vi "反控仪器单参数通用.vi"(8 "错误输入（无错误）":errorcluster, 9 "参数":string, 10 "value float":sgl, 11 "chose":string="写入") -> (0 "错误输出":errorcluster, 3 "超时？":bool)   [LabVIEW 2016]
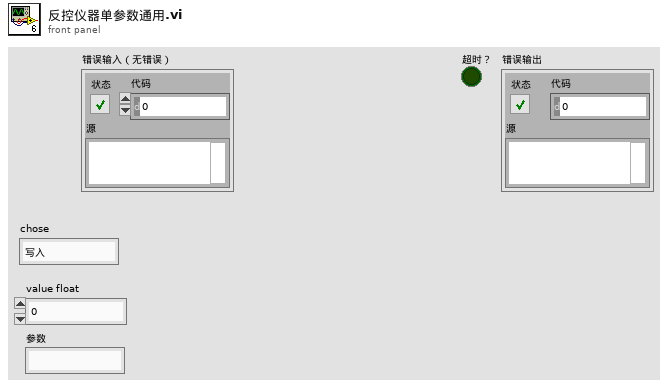
[diagram p1: front panel]
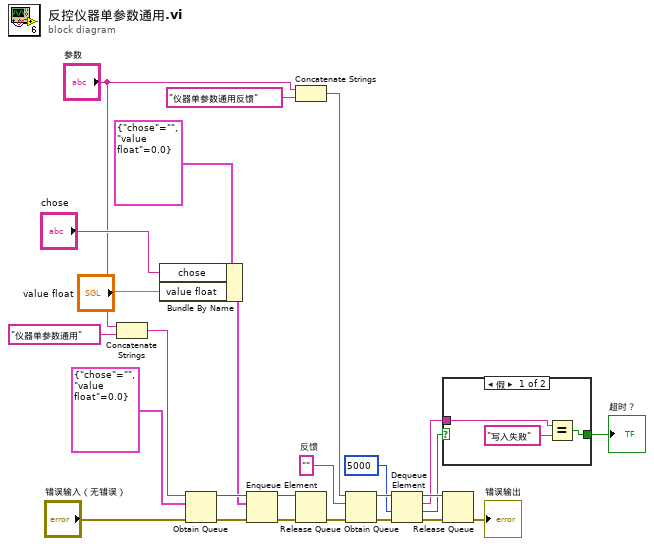
[diagram p0: block diagram]
diagram:
  w26 = ""  # 反馈
  n1 = Concatenate Strings("参数", "仪器单参数通用" ("名称（未命名）")) -> (w2:string)
  n2 = Bundle By Name(cluster=cluster{"chose":string, "value float":dbl} {"chose"="", "value float"=0.0}, "chose"="chose", "value float"="value float") -> (w20:cluster{"chose":string, "value float":dbl})
  n3 = Obtain Queue(name (unnamed)=w2, element data type=cluster{"chose":string, "value float":dbl} {"chose"="", "value float"=0.0}, error in (no error)="错误输入（无错误）") -> (queue out=w25:refnum<queue>, error out=w24:errorcluster)  [unwired: 2 in, 1 out]
  n4 = Enqueue Element(queue=w25, element=w20, error in (no error)=w24) -> (queue out=w19:refnum<queue>, error out=w18:errorcluster)  [unwired: 1 in, 1 out]
  n5 = Concatenate Strings("参数", "仪器单参数通用反馈" ("名称（未命名）")) -> (w3:string)
  n6 = Release Queue(queue=w19, error in (no error)=w18) -> (error out=w17:errorcluster)  [unwired: 1 in, 2 out]
  n7 = Obtain Queue(name (unnamed)=w3, element data type=w26, error in (no error)=w17) -> (queue out=w16:refnum<queue>, error out=w15:errorcluster)  [unwired: 2 in, 1 out]
  n8 = Dequeue Element(queue=w16, timeout in ms (-1)=5000 ("超时毫秒(-1)"), error in (no error)=w15) -> (queue out=w12:refnum<queue>, element=w11:string, timed out?=w10:bool, error out=w13:errorcluster)
  n9 = case shown="假" w10 {
    selector: w10 -> [_ w30]
    tunnel: w11 -> [w28 _]
    tunnel: [w27 w30] -> w9
    frame False {
      n10 = Equal?(x=w28, y="写入失败") -> (x = y?=w27:bool)
    }
    frame True {
    }
  }
  "超时？" <- w9
  n11 = Release Queue(queue=w12, error in (no error)=w13) -> (error out=→"错误输出":errorcluster)  [unwired: 1 in, 2 out]
